vi "Read Process Name.vi"(11 "Process In":refnum<class "Process.lvclass">) -> (2 "Process Name":string, 3 "Process Out":refnum<class "Process.lvclass">)   [LabVIEW 2020, in "Process.lvclass"]
uses:
  Process.lvclass
  Process.lvclass/Process.ctl
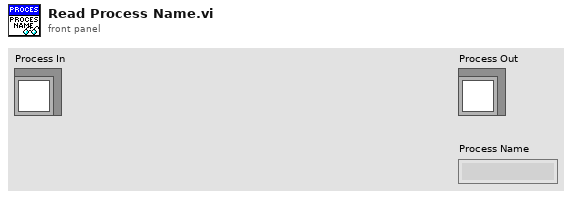
[diagram p1: front panel]
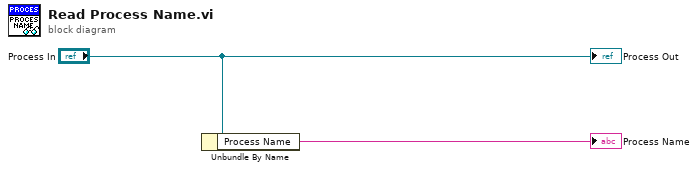
[diagram p0: block diagram]
diagram:
  n1 = Unbundle By Name("Process In") -> ("Process Name"=→"Process Name":string)
  "Process Out" <- "Process In"
